vi "QueuedStateHandler.vi"(8 "error in (no error)":errorcluster, 10 "Array":T1[](array[typedef]), 11 "queue out":refnum<queue>) -> (0 "error out":errorcluster)   [LabVIEW 2020]
uses:
  Controls/SprinklerStates.ctl
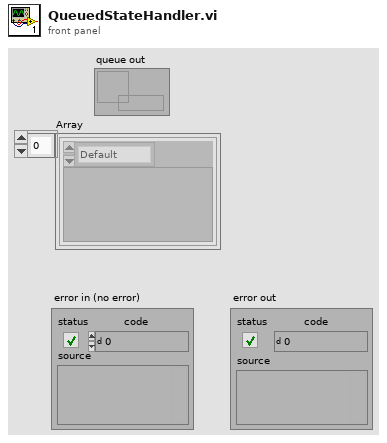
[diagram p1: front panel]
types:
  T1 = typedef "SprinklerStates.ctl" = cluster{enum16{"Default", "Init", "Setup", "Start", "Stop"}, variant}
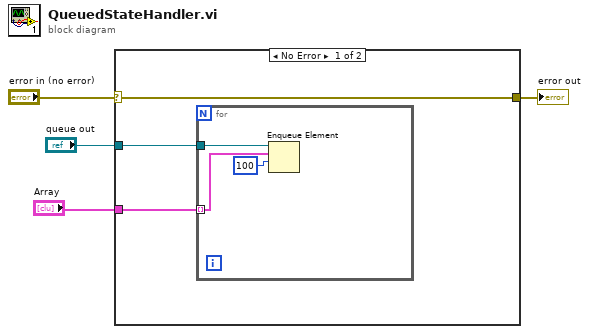
[diagram p0: block diagram]
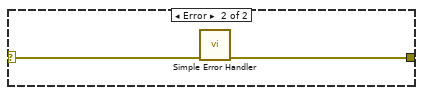
[diagram p2: hidden frame]
diagram:
  n1 = case shown="No Error" "error in (no error)" {
    selector: "error in (no error)" -> [w6 w12]
    tunnel: [w6 w11] -> w3
    tunnel: "queue out" -> [w7 _]
    tunnel: "Array" -> [w5 _]
    frame No Error {
      n2 = for {
        tunnel: w7 -> [w10]
        tunnel: w5 -> [w8] mode=indexing
        n3 = Enqueue Element(queue=w10, element=w8, timeout in ms (-1)=100) -> ()  [unwired: 1 in, 3 out]
      }
    }
    frame Error {
      n4 = call <vilib>:"Simple Error Handler.vi"("error in (no error)"=w12) -> ("error out"=w11:errorcluster)  [unwired: 4 in, 4 out]
    }
  }
  "error out" <- w3
